vi "BRig_dataExp_T_RewardPost.vi"() -> (2 "output_T_RewardPost":i32)   [LabVIEW 2014]
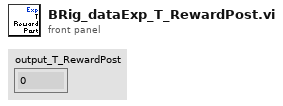
[diagram p1: front panel]
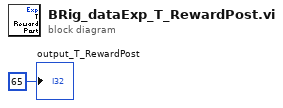
[diagram p0: block diagram]
diagram:
  "output_T_RewardPost" <- 65 ("output_iBlock")
